vi "NameData_Array Number determine.vi"(8 "Error":errorcluster, 9 "Dim Sizes":u32[](array[numeric]), 11 "Row Index":i32) -> (0 "Error Out":errorcluster, 3 "Row Numbers Out":u32[](array[numeric]))   [LabVIEW 2015]
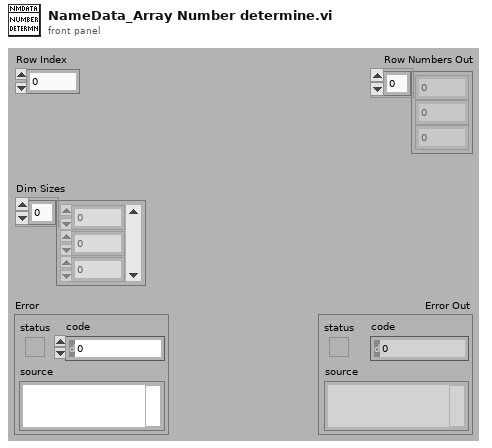
[diagram p1: front panel]
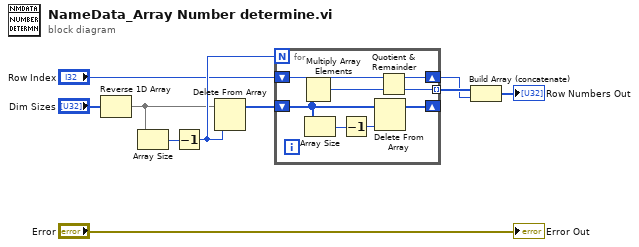
[diagram p0: block diagram]
diagram:
  n1 = Reverse 1D Array(array="Dim Sizes") -> (reversed array=w2:u32[])
  n2 = Array Size(array=w2) -> (size(s)=w8:i32)
  n3 = Decrement(x=w8) -> (x-1=w5:i32)
  n4 = Delete From Array(array=w2, index=w5) -> (array with subset deleted=w9:u32[])  [unwired: 1 in, 1 out]
  n5 = for {
    N: w5 -> [_]
    tunnel: [w17] -> w10 mode=indexing
    shift-right: [w12] -> w4
    shift-left: "Row Index" -> [w18]
    shift-right: [w16] -> _
    shift-left: w9 -> [w15]
    n6 = Multiply Array Elements(1:w15) -> (0:w11:u32)
    n7 = Array Size(array=w15) -> (size(s)=w14:i32)
    n8 = Decrement(x=w14) -> (x-1=w13:i32)
    n9 = Delete From Array(array=w15, index=w13) -> (array with subset deleted=w16:u32[])  [unwired: 1 in, 1 out]
    n10 = Quotient & Remainder(x=w18, y=w11) -> (x-y*floor(x/y)=w12:u32, floor(x/y)=w17:u32)
  }
  n11 = Build Array (concatenate)(w10, w4) -> (→"Row Numbers Out":u32[])
  "Error Out" <- "Error"
